vi "PictureControlGUIForMissingClasses.vi"() -> ()   [LabVIEW 2016]
uses:
  <vilib>/picture/picture.llb/imagedata.ctl
  <vilib>/Utility/miscctls.llb/LVFontTypeDef.ctl
  <vilib>/Utility/miscctls.llb/LVBoundsTypeDef.ctl
panel:
  in  "Items":T1(array[cluster])=[{"Item"="IDisposne", "Options"=["Select action to handle missing type", "Create stub code as class", "Create stub code as interface by aggregation", "Create stub code as interface by VI Serevr", "Remove dependency to this type"], "Icons"=[enum."?", enum."Add", enum."Add", enum."Add", enum."Delete"], "InitialIndex"=0}, {"Item"="IInterafceXXX", "Options"=["Select action to handle missing type", "Create stub code as class", "Create stub code as interface by VI Serevr", "Remove dependency to this type"], "Icons"=[enum."?", enum."Add", enum."Add", enum."Delete"], "InitialIndex"=1}, {"Item"="Something Something", "Options"=["Select action to handle missing type", "Create stub code as class", "Remove dependency to this type"], "Icons"=[enum."?", enum."Add", enum."Delete"], "InitialIndex"=2}, {"Item"="Something Something", "Options"=["Select action to handle missing type", "Create stub code as class", "Remove dependency to this type"], "Icons"=[enum."?", enum."Add", enum."Delete"], "InitialIndex"=2}, {"Item"="Something Something", "Options"=["Select action to handle missing type", "Create stub code as class", "Remove dependency to this type"], "Icons"=[enum."?", enum."Add", enum."Delete"], "InitialIndex"=2}, {"Item"="Something Something", "Options"=["Select action to handle missing type", "Create stub code as class", "Remove dependency to this type"], "Icons"=[enum."?", enum."Add", enum."Delete"], "InitialIndex"=2}, {"Item"="Something Something", "Options"=["Select action to handle missing type", "Create stub code as class", "Remove dependency to this type"], "Icons"=[enum."?", enum."Add", enum."Delete"], "InitialIndex"=2}, {"Item"="Something Something", "Options"=["Select action to handle missing type", "Create stub code as class", "Remove dependency to this type"], "Icons"=[enum."?", enum."Add", enum."Delete"], "InitialIndex"=2}]
  out "Mouse Position":cluster{"X":i32, "Y":i32}={"X"=267, "Y"=20}
  in  "Ring":u16(ring)=2 items=["Select action to handle missing type", "Create stub code as class", "Remove dependency to this type"]
  out "Picture":picture caption="Missing Classes and types"
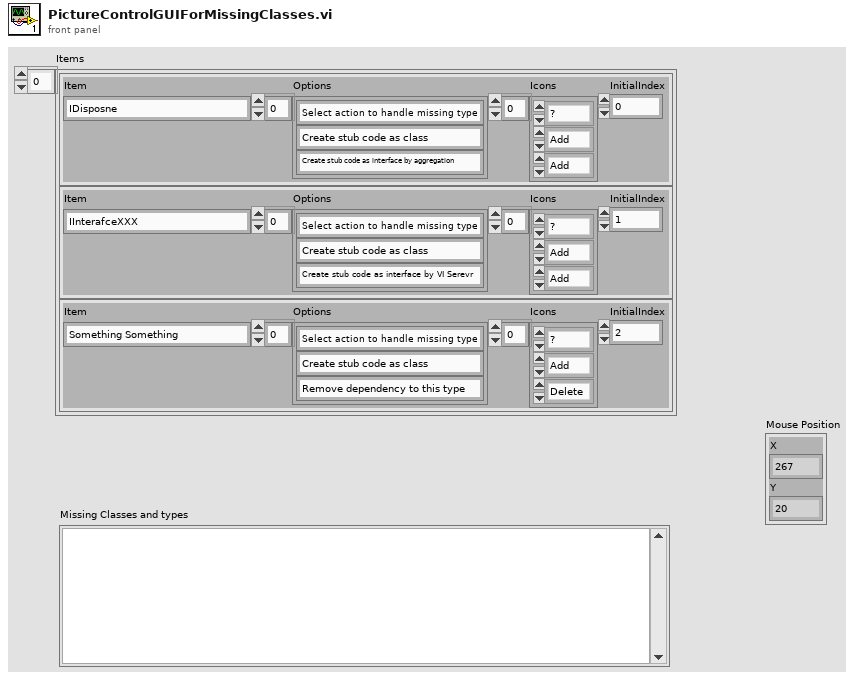
[diagram p1: front panel]
types:
  T1 = cluster{"Item":string, "Options":string[], "Icons":enum16{"?", "Add", "Delete"}[], "InitialIndex":i32}[]
  T2 = typedef "imagedata.ctl" = cluster{"image type":i32, "image depth":i32, "image":u8[], "mask":u8[], "colors":u32[], "Rectangle":cluster{"left":i16, "top":i16, "right":i16, "bottom":i16}}
  T3 = cluster{"ShowRing":bool, "Rectangle":cluster{"left":i16, "top":i16, "right":i16, "bottom":i16}, "IndexOffset":i32, "Row":i32, "Y-Distance":i32, "Selected":i32[], "Font":enum16{"User-specified Font", "Application Font", "System Font", "Dialog Font"}, "UserFont":cluster{"Font Name:":string, "Size":i16, "Strikeout?":bool, "Italic?":bool, "Underline?":bool, "Outline?":bool, "Shadow?":bool, "Bold?":bool}, "VerGap":i32, "HorGap":i32, "XStart2":i32, "XStart1":i32, "Rectangles":cluster{"left":i16, "top":i16, "right":i16, "bottom":i16}[], "VerticalRows":i32, "YStart":i32}
  T4 = typedef "LVFontTypeDef.ctl" = cluster{"Font Name":string, "Size":u16, "Bold":bool, "Italic":bool, "Underline":bool, "Strikeout":bool, "Color":u32}
  T5 = cluster{"left":i16, "top":i16, "right":i16, "bottom":i16}
  T6 = typedef "LVBoundsTypeDef.ctl" = cluster{"Width":u32, "Height":u32}
  T7 = cluster{"Font Name:":string, "Size":i16, "Strikeout?":bool, "Italic?":bool, "Underline?":bool, "Outline?":bool, "Shadow?":bool, "Bold?":bool}
  T8 = enum16{"User-specified Font", "Application Font", "System Font", "Dialog Font"}
  T9 = typedef "LVMouseTypeDef.ctl" = cluster{"Mouse Position":cluster{"X":i32, "Y":i32}, "Mouse Modifiers":cluster{"Button Down":bool, "Shift Mod":bool, "Menu Mod":bool, "Option Mod":bool}}
  T10 = cluster{"left":i16, "top":i16, "right":i16, "bottom":i16}[]
  T11 = cluster{"Item":string, "Options":string[], "Icons":enum16{"?", "Add", "Delete"}[], "InitialIndex":i32}
  T12 = typedef "LVRectTypeDef.ctl" = cluster{"Left":i16, "Top":i16, "Right":i16, "Bottom":i16}
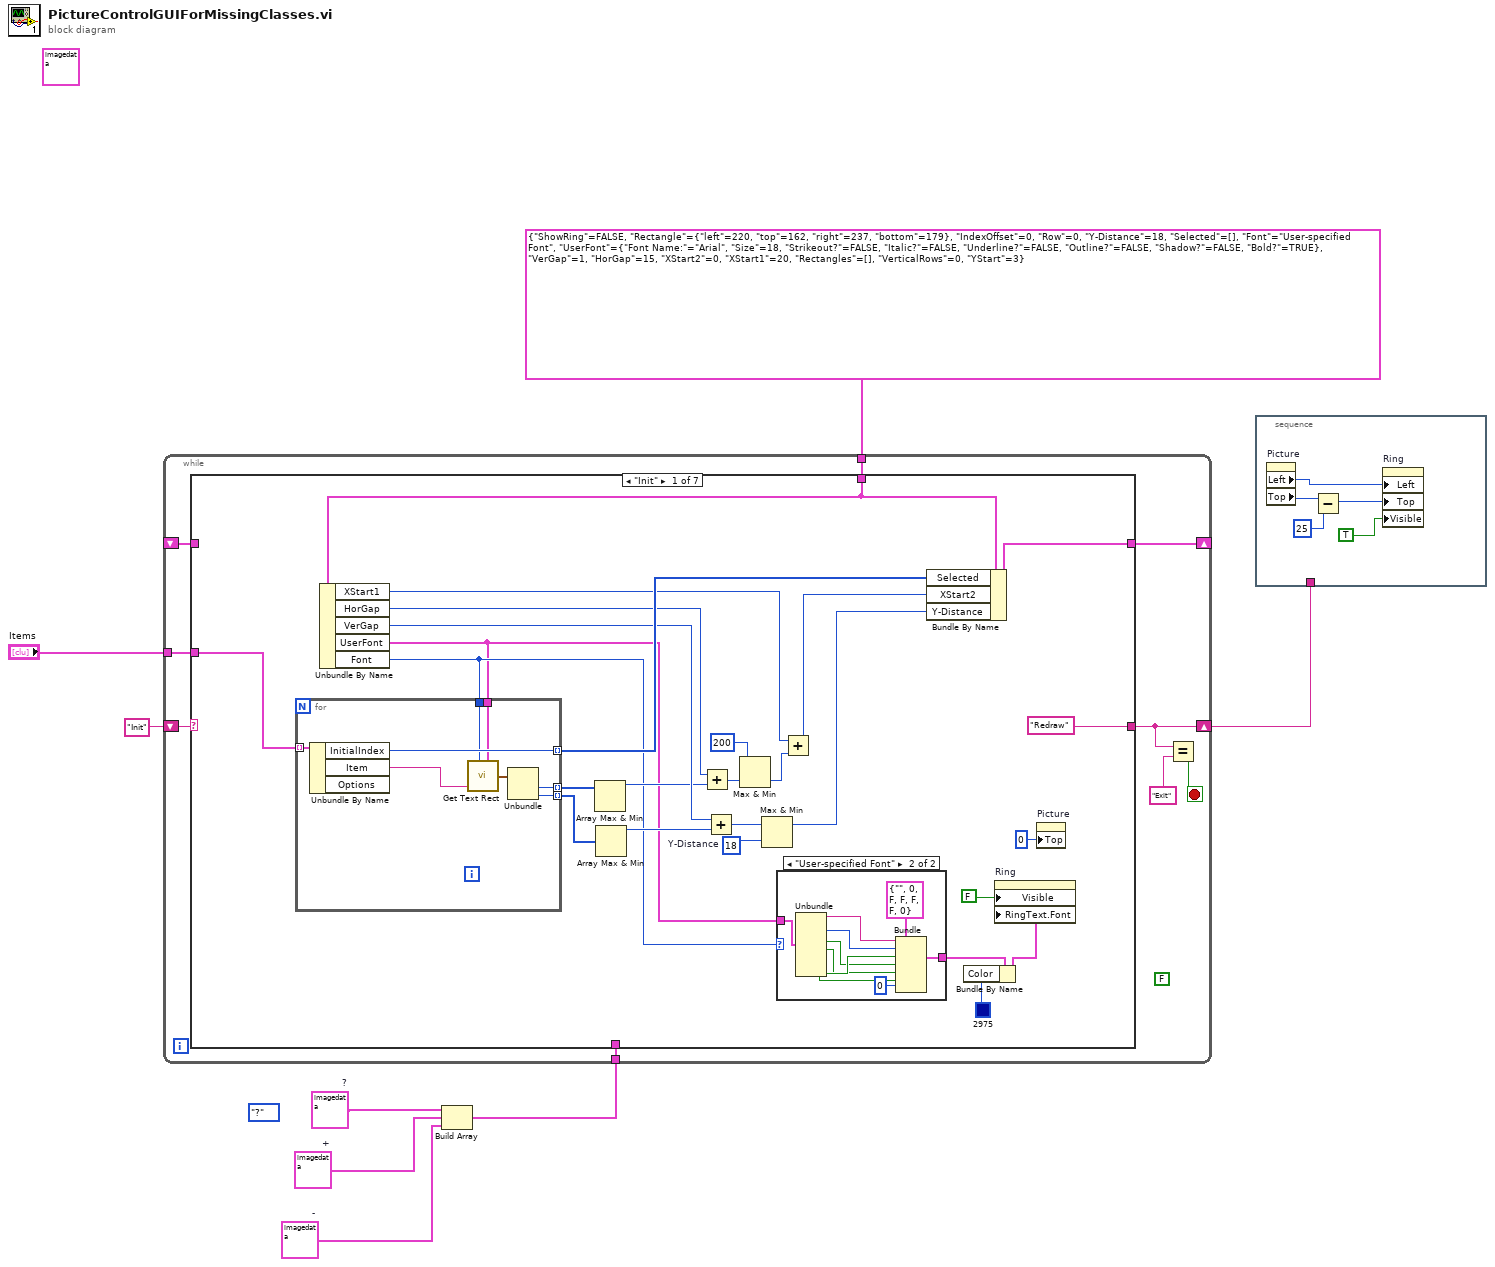
[diagram p0: block diagram]
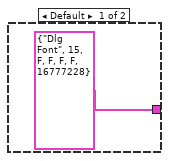
[diagram p2: hidden frame]
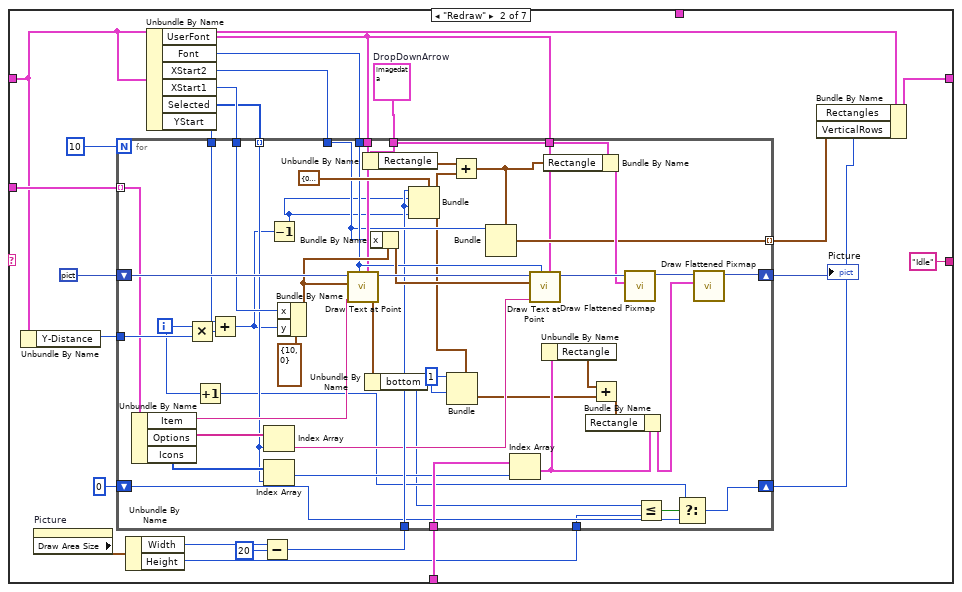
[diagram p3: hidden frame]
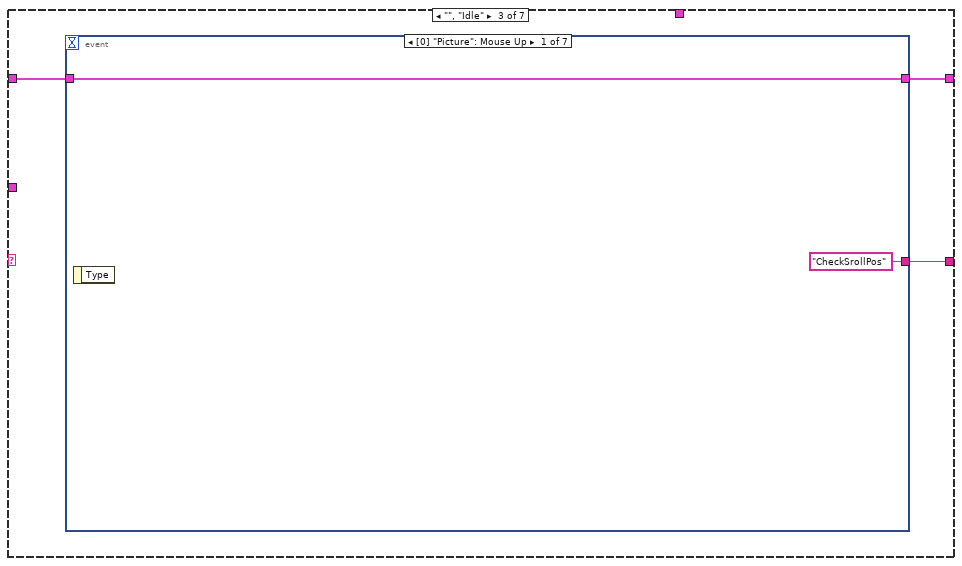
[diagram p4: hidden frame]
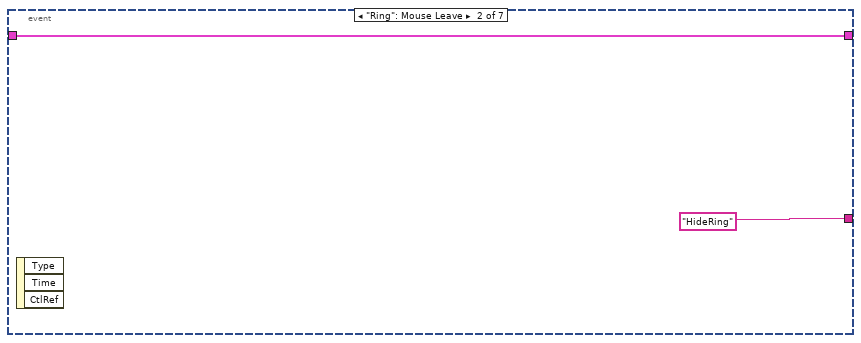
[diagram p5: hidden frame]
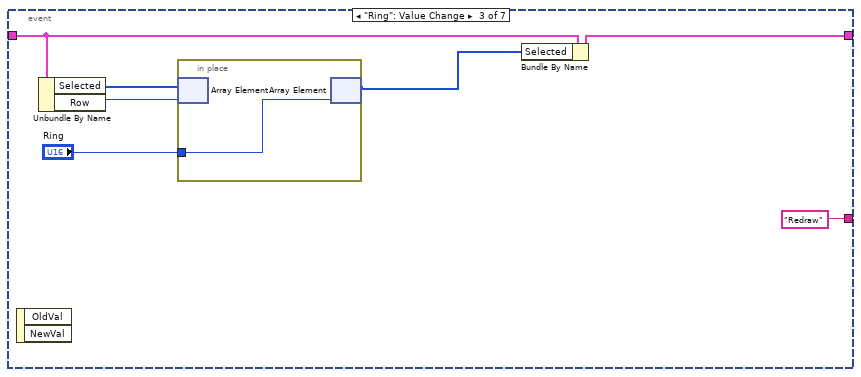
[diagram p6: hidden frame]
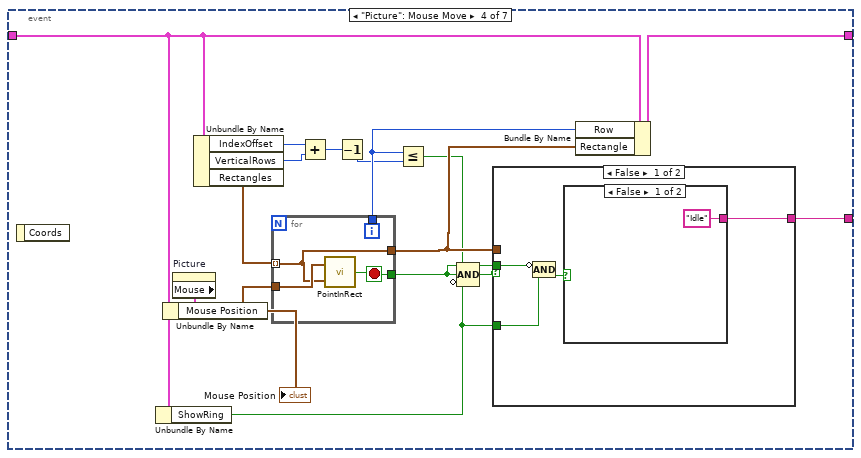
[diagram p7: hidden frame]
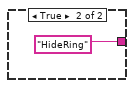
[diagram p8: hidden frame]
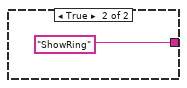
[diagram p9: hidden frame]
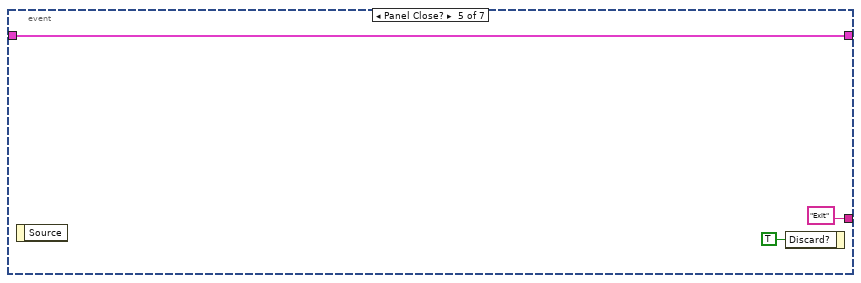
[diagram p10: hidden frame]
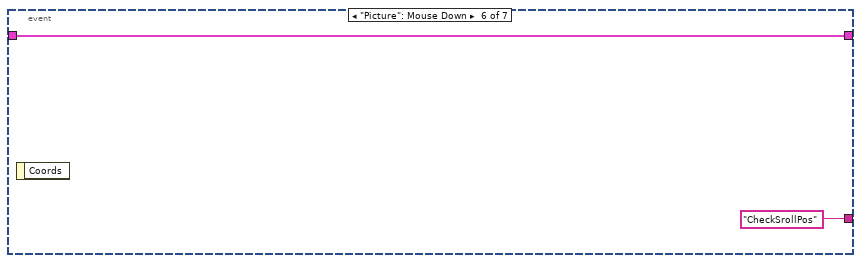
[diagram p11: hidden frame]
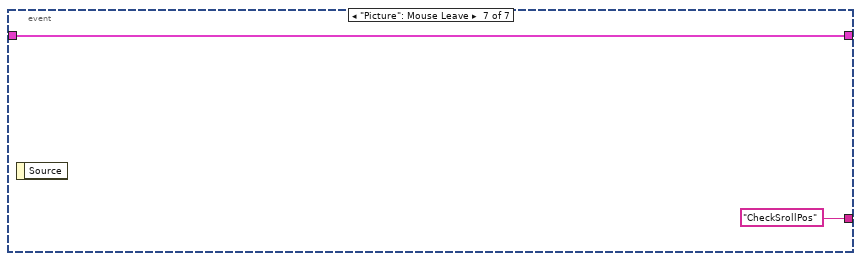
[diagram p12: hidden frame]
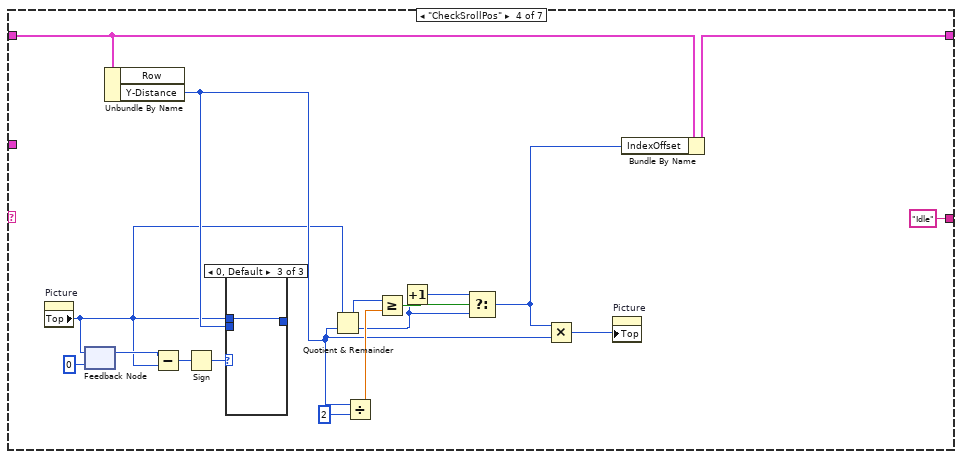
[diagram p13: hidden frame]
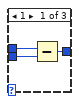
[diagram p14: hidden frame]
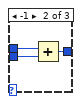
[diagram p15: hidden frame]
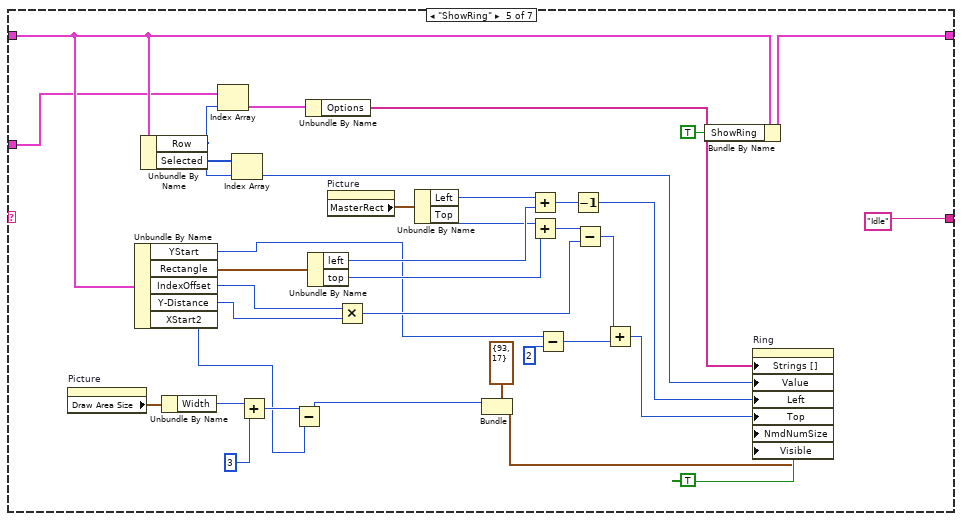
[diagram p16: hidden frame]
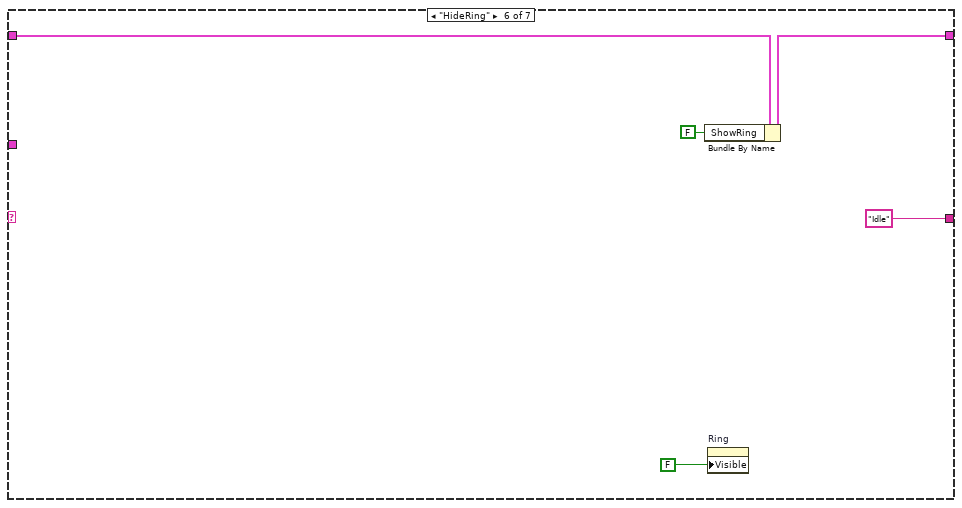
[diagram p17: hidden frame]
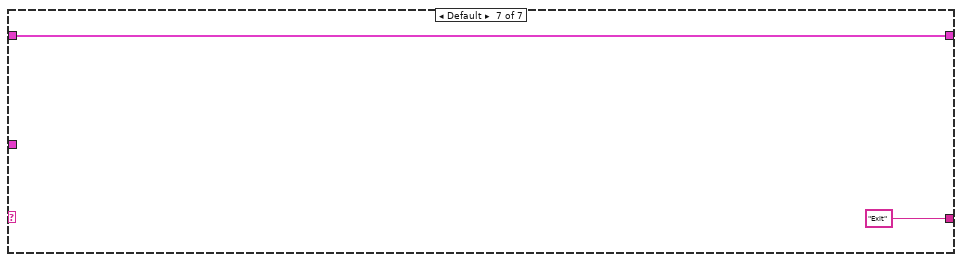
[diagram p18: hidden frame]
diagram:
  (unwired) enum16{"?", "Add", "Delete"}."?" ("element")
  w3 = T2 {"image type"=0, "image depth"=32, "image"=array[1024 elements], "mask"=[0, 0, 15, 224, 63, 248, 127, 252, 127, 252, 255, 254, 255, 254, 255, 254, 255, 254, 255, 254, 255, 254, 255, 254, 127, 252, 127, 252, 63, 248, 15, 224], "colors"=[], "Rectangle"={"left"=0, "top"=0, "right"=16, "bottom"=16}}  # ?
  w1 = T2 {"image type"=0, "image depth"=32, "image"=[0, 0, 0, 0, 0, 0, 0, 0, 78, 142, 77, 90, 2, 148, 148, 147, 0, 0, 0, 0, 0, 0, 0, 0, 0, 0, 0, 0, 0, 0, 0, 0, 0, 0, 0, 0, 0, 0, 0, 0, 0, 0, 0, 0, 48, 145, 103, 111, 3, 148, 145, 146, 0, 0, 0, 0, 0, 0, 0, 0, 0, 0, 0, 0, 0, 0, 0, 0, 113, 246, 155, 172, 255, 238, 54, 90, 164, 243, 121, 144, 0, 0, 0, 0, 0, 0, 0, 0, 0, 0, 0, 0, 0, 0, 0, 0, 0, 0, 0, 0, 0, 0, 0, 0, 114, 247, 158, 175, 255, 238, 55, 91, 247, 238, 61, 95, 190, 242, 101, 128, 55, 251, 205, 215, 0, 0, 0, 0, 37, 251, 214, 220, 252, 236, 52, 88, 255, 237, 57, 92, 255, 235, 54, 90, 150, 242, 130, 151, 0, 0, 0, 0, 0, 0, 0, 0, 0, 0, 0, 0, 0, 0, 0, 0, 64, 249, 199, 209, 253, 236, 55, 90, 254, 235, 56, 91, 255, 236, 54, 90, 127, 244, 146, 165, 0, 0, 0, 0, 0, 0, 0, 0, 0, 0, 0, 0, 64, 249, 193, 203, 240, 236, 60, 95, 255, 237, 57, 92, 255, 236, 55, 90, 136, 243, 141, 161, 0, 0, 0, 0, 0, 0, 0, 0, 25, 252, 231, 235, 235, 237, 66, 99, 255, 236, 57, 92, 255, 236, 54, 90, 118, 244, 150, 168, 0, 0, 0, 0, 0, 0, 0, 0, 0, 0, 0, 0, 0, 0, 0, 0, 0, 0, 0, 0, 39, 251, 215, 222, 224, 237, 70, 103, 255, 236, 57, 92, 255, 235, 53, 89, 121, 244, 152, 170, 1, 254, 253, 254, 201, 239, 91, 120, 254, 235, 56, 91, 255, 236, 55, 90, 121, 244, 150, 168, 0, 0, 0, 0, 0, 0, 0, 0, 0, 0, 0, 0, 0, 0, 0, 0, 0, 0, 0, 0, 0, 0, 0, 0, 0, 0, 0, 0, 20, 252, 233, 236, 204, 238, 86, 115, 255, 236, 57, 92, 255, 236, 55, 91, 194, 239, 93, 122, 255, 236, 56, 92, 255, 236, 55, 90, 133, 243, 143, 163, 0, 0, 0, 0, 0, 0, 0, 0, 0, 0, 0, 0, 0, 0, 0, 0, 0, 0, 0, 0, 0, 0, 0, 0, 0, 0, 0, 0, 0, 0, 0, 0, 0, 0, 0, 0, 12, 253, 243, 245, 210, 238, 83, 114, 255, 236, 57, 92, 254, 235, 56, 91, 255, 236, 56, 92, 149, 242, 132, 153, 0, 0, 0, 0, 0, 0, 0, 0, 0, 0, 0, 0, 0, 0, 0, 0, 0, 0, 0, 0, 0, 0, 0, 0, 0, 0, 0, 0, 0, 0, 0, 0, 0, 0, 0, 0, 0, 0, 0, 0, 0, 0, 0, 0, 78, 248, 186, 198, 255, 236, 55, 91, 255, 237, 58, 93, 253, 236, 55, 90, 39, 251, 220, 226, 0, 0, 0, 0, 0, 0, 0, 0, 0, 0, 0, 0, 0, 0, 0, 0, 0, 0, 0, 0, 0, 0, 0, 0, 0, 0, 0, 0, 0, 0, 0, 0, 0, 0, 0, 0, 0, 0, 0, 0, 11, 253, 244, 245, 222, 237, 74, 105, 254, 236, 56, 92, 253, 236, 56, 91, 255, 236, 57, 92, 210, 238, 85, 116, 5, 254, 250, 250, 0, 0, 0, 0, 0, 0, 0, 0, 0, 0, 0, 0, 0, 0, 0, 0, 0, 0, 0, 0, 0, 0, 0, 0, 0, 0, 0, 0, 0, 0, 0, 0, 0, 0, 0, 0, 167, 241, 117, 142, 255, 236, 55, 91, 179, 240, 108, 134, 139, 244, 138, 159, 255, 236, 56, 91, 255, 236, 56, 91, 147, 243, 132, 153, 0, 0, 0, 0, 0, 0, 0, 0, 0, 0, 0, 0, 0, 0, 0, 0, 0, 0, 0, 0, 0, 0, 0, 0, 0, 0, 0, 0, 0, 0, 0, 0, 100, 247, 169, 184, 255, 236, 55, 90, 255, 235, 54, 90, 54, 250, 206, 215, 6, 253, 248, 249, 227, 237, 71, 103, 254, 235, 56, 91, 255, 236, 54, 90, 77, 248, 188, 200, 0, 0, 0, 0, 0, 0, 0, 0, 0, 0, 0, 0, 0, 0, 0, 0, 0, 0, 0, 0, 0, 0, 0, 0, 40, 251, 219, 224, 247, 236, 57, 92, 255, 236, 57, 92, 185, 240, 103, 129, 0, 0, 0, 0, 0, 0, 0, 0, 100, 246, 164, 180, 255, 236, 56, 91, 255, 236, 57, 92, 238, 237, 64, 98, 25, 252, 232, 236, 0, 0, 0, 0, 0, 0, 0, 0, 0, 0, 0, 0, 0, 0, 0, 0, 4, 254, 250, 251, 211, 238, 83, 113, 254, 235, 56, 91, 255, 236, 54, 90, 56, 250, 206, 214, 0, 0, 0, 0, 0, 0, 0, 0, 4, 254, 247, 249, 228, 237, 68, 100, 255, 237, 57, 92, 254, 235, 56, 91, 193, 239, 96, 125, 0, 0, 0, 0, 0, 0, 0, 0, 0, 0, 0, 0, 0, 0, 0, 0, 139, 244, 137, 157, 255, 237, 55, 91, 255, 237, 56, 92, 188, 229, 93, 119, 0, 0, 0, 0, 0, 0, 0, 0, 0, 0, 0, 0, 0, 0, 0, 0, 105, 246, 160, 177, 255, 236, 55, 90, 255, 236, 56, 92, 255, 236, 54, 90, 127, 244, 148, 166, 0, 0, 0, 0, 0, 0, 0, 0, 26, 246, 224, 228, 199, 228, 84, 112, 200, 227, 87, 114, 201, 227, 85, 113, 57, 237, 196, 204, 0, 0, 0, 0, 0, 0, 0, 0, 0, 0, 0, 0, 0, 0, 0, 0, 7, 254, 247, 249, 171, 231, 108, 133, 170, 241, 120, 144, 167, 239, 120, 143, 162, 235, 117, 140, 17, 241, 227, 230, 0, 0, 0, 0, 0, 0, 0, 0, 0, 0, 0, 0, 0, 0, 0, 0, 0, 0, 0, 0, 0, 0, 0, 0, 0, 0, 0, 0, 0, 0, 0, 0, 0, 0, 0, 0, 0, 0, 0, 0, 0, 0, 0, 0, 0, 0, 0, 0, 0, 0, 0, 0, 0, 0, 0, 0, 0, 0, 0, 0, 0, 0, 0, 0, 0, 0, 0, 0], "mask"=[0, 0, 48, 28, 120, 60, 60, 112, 28, 224, 15, 224, 7, 192, 3, 128, 7, 192, 15, 224, 12, 224, 28, 112, 56, 120, 120, 60, 112, 60, 0, 0], "colors"=[], "Rectangle"={"left"=0, "top"=0, "right"=16, "bottom"=16}}  # -
  w2 = T2 {"image type"=0, "image depth"=32, "image"=[0, 0, 0, 0, 0, 0, 0, 0, 0, 0, 0, 0, 0, 0, 0, 0, 0, 0, 0, 0, 255, 0, 173, 0, 255, 0, 173, 0, 255, 0, 173, 0, 255, 0, 173, 0, 255, 0, 173, 0, 0, 0, 0, 0, 0, 0, 0, 0, 0, 0, 0, 0, 0, 0, 0, 0, 0, 0, 0, 0, 0, 0, 0, 0, 0, 0, 0, 0, 0, 0, 0, 0, 0, 0, 0, 0, 0, 0, 0, 0, 0, 0, 0, 0, 255, 0, 173, 0, 255, 0, 173, 0, 255, 0, 173, 0, 255, 0, 173, 0, 255, 0, 173, 0, 255, 106, 100, 106, 0, 0, 0, 0, 0, 0, 0, 0, 0, 0, 0, 0, 0, 0, 0, 0, 0, 0, 0, 0, 0, 0, 0, 0, 0, 0, 0, 0, 0, 0, 0, 0, 0, 0, 0, 0, 0, 0, 0, 0, 255, 0, 173, 0, 255, 0, 173, 0, 255, 0, 173, 0, 255, 0, 173, 0, 255, 0, 173, 0, 255, 106, 100, 106, 0, 0, 0, 0, 0, 0, 0, 0, 0, 0, 0, 0, 0, 0, 0, 0, 0, 0, 0, 0, 0, 0, 0, 0, 0, 0, 0, 0, 0, 0, 0, 0, 0, 0, 0, 0, 0, 0, 0, 0, 255, 0, 173, 0, 255, 0, 173, 0, 255, 0, 173, 0, 255, 0, 173, 0, 255, 0, 173, 0, 255, 106, 100, 106, 0, 0, 0, 0, 0, 0, 0, 0, 0, 0, 0, 0, 0, 0, 0, 0, 0, 0, 0, 0, 0, 0, 0, 0, 0, 0, 0, 0, 0, 0, 0, 0, 0, 0, 0, 0, 0, 0, 0, 0, 255, 0, 173, 0, 255, 0, 173, 0, 255, 0, 173, 0, 255, 0, 173, 0, 255, 0, 173, 0, 255, 106, 100, 106, 0, 0, 0, 0, 0, 0, 0, 0, 0, 0, 0, 0, 0, 0, 0, 0, 0, 0, 0, 0, 255, 0, 173, 0, 255, 0, 173, 0, 255, 0, 173, 0, 255, 0, 173, 0, 255, 0, 173, 0, 255, 0, 173, 0, 255, 0, 173, 0, 255, 0, 173, 0, 255, 0, 173, 0, 255, 0, 173, 0, 255, 0, 173, 0, 255, 0, 173, 0, 255, 0, 173, 0, 255, 0, 173, 0, 255, 0, 173, 0, 0, 0, 0, 0, 255, 0, 173, 0, 255, 0, 173, 0, 255, 0, 173, 0, 255, 0, 173, 0, 255, 0, 173, 0, 255, 0, 173, 0, 255, 0, 173, 0, 255, 0, 173, 0, 255, 0, 173, 0, 255, 0, 173, 0, 255, 0, 173, 0, 255, 0, 173, 0, 255, 0, 173, 0, 255, 0, 173, 0, 255, 0, 173, 0, 255, 106, 100, 106, 255, 0, 173, 0, 255, 0, 173, 0, 255, 0, 173, 0, 255, 0, 173, 0, 255, 0, 173, 0, 255, 0, 173, 0, 255, 0, 173, 0, 255, 0, 173, 0, 255, 0, 173, 0, 255, 0, 173, 0, 255, 0, 173, 0, 255, 0, 173, 0, 255, 0, 173, 0, 255, 0, 173, 0, 255, 0, 173, 0, 255, 106, 100, 106, 255, 0, 173, 0, 255, 0, 173, 0, 255, 0, 173, 0, 255, 0, 173, 0, 255, 0, 173, 0, 255, 0, 173, 0, 255, 0, 173, 0, 255, 0, 173, 0, 255, 0, 173, 0, 255, 0, 173, 0, 255, 0, 173, 0, 255, 0, 173, 0, 255, 0, 173, 0, 255, 0, 173, 0, 255, 0, 173, 0, 255, 106, 100, 106, 255, 0, 173, 0, 255, 0, 173, 0, 255, 0, 173, 0, 255, 0, 173, 0, 255, 0, 173, 0, 255, 0, 173, 0, 255, 0, 173, 0, 255, 0, 173, 0, 255, 0, 173, 0, 255, 0, 173, 0, 255, 0, 173, 0, 255, 0, 173, 0, 255, 0, 173, 0, 255, 0, 173, 0, 255, 0, 173, 0, 255, 106, 100, 106, 0, 0, 0, 0, 255, 106, 100, 106, 255, 106, 100, 106, 255, 106, 100, 106, 255, 106, 100, 106, 255, 0, 173, 0, 255, 0, 173, 0, 255, 0, 173, 0, 255, 0, 173, 0, 255, 0, 173, 0, 255, 106, 100, 106, 255, 106, 100, 106, 255, 106, 100, 106, 255, 106, 100, 106, 255, 106, 100, 106, 255, 106, 100, 106, 0, 0, 0, 0, 0, 0, 0, 0, 0, 0, 0, 0, 0, 0, 0, 0, 0, 0, 0, 0, 255, 0, 173, 0, 255, 0, 173, 0, 255, 0, 173, 0, 255, 0, 173, 0, 255, 0, 173, 0, 255, 106, 100, 106, 0, 0, 0, 0, 0, 0, 0, 0, 0, 0, 0, 0, 0, 0, 0, 0, 0, 0, 0, 0, 0, 0, 0, 0, 0, 0, 0, 0, 0, 0, 0, 0, 0, 0, 0, 0, 0, 0, 0, 0, 255, 0, 173, 0, 255, 0, 173, 0, 255, 0, 173, 0, 255, 0, 173, 0, 255, 0, 173, 0, 255, 106, 100, 106, 0, 0, 0, 0, 0, 0, 0, 0, 0, 0, 0, 0, 0, 0, 0, 0, 0, 0, 0, 0, 0, 0, 0, 0, 0, 0, 0, 0, 0, 0, 0, 0, 0, 0, 0, 0, 0, 0, 0, 0, 255, 0, 173, 0, 255, 0, 173, 0, 255, 0, 173, 0, 255, 0, 173, 0, 255, 0, 173, 0, 255, 106, 100, 106, 0, 0, 0, 0, 0, 0, 0, 0, 0, 0, 0, 0, 0, 0, 0, 0, 0, 0, 0, 0, 0, 0, 0, 0, 0, 0, 0, 0, 0, 0, 0, 0, 0, 0, 0, 0, 0, 0, 0, 0, 255, 0, 173, 0, 255, 0, 173, 0, 255, 0, 173, 0, 255, 0, 173, 0, 255, 0, 173, 0, 255, 106, 100, 106, 0, 0, 0, 0, 0, 0, 0, 0, 0, 0, 0, 0, 0, 0, 0, 0, 0, 0, 0, 0, 0, 0, 0, 0, 0, 0, 0, 0, 0, 0, 0, 0, 0, 0, 0, 0, 0, 0, 0, 0, 0, 0, 0, 0, 255, 106, 100, 106, 255, 106, 100, 106, 255, 106, 100, 106, 255, 106, 100, 106, 255, 106, 100, 106, 0, 0, 0, 0, 0, 0, 0, 0, 0, 0, 0, 0, 0, 0, 0, 0, 0, 0, 0, 0], "mask"=[7, 192, 7, 224, 7, 224, 7, 224, 7, 224, 255, 254, 255, 255, 255, 255, 255, 255, 255, 255, 127, 255, 7, 224, 7, 224, 7, 224, 7, 224, 3, 224], "colors"=[], "Rectangle"={"left"=0, "top"=0, "right"=16, "bottom"=16}}  # +
  (unwired) T2 {"image type"=0, "image depth"=32, "image"=array[1156 elements], "mask"=[255, 255, 128, 0, 255, 255, 128, 0, 255, 255, 128, 0, 255, 255, 128, 0, 255, 255, 128, 0, 255, 255, 128, 0, 255, 255, 128, 0, 255, 255, 128, 0, 255, 255, 128, 0, 255, 255, 128, 0, 255, 255, 128, 0, 255, 255, 128, 0, 255, 255, 128, 0, 255, 255, 128, 0, 255, 255, 128, 0, 255, 255, 128, 0, 255, 255, 128, 0], "colors"=[], "Rectangle"={"left"=0, "top"=0, "right"=17, "bottom"=17}} ("image data")
  n1 = Build Array(w3, w2, w1) -> (w4:T2[])
  n2 = while {
    shift-right: [w14] -> w5
    shift-left: "Init" ("format string") -> [w17]
    shift-right: [w16] -> _
    shift-left: _ -> [w15]
    tunnel: "Items" -> [w11]
    tunnel: T3 {"ShowRing"=FALSE, "Rectangle"={"left"=220, "top"=162, "right"=237, "bottom"=179}, "IndexOffset"=0, "Row"=0, "Y-Distance"=18, "Selected"=[], "Font"=enum."User-specified Font", "UserFont"={"Font Name:"="Arial", "Size"=18, "Strikeout?"=FALSE, "Italic?"=FALSE, "Underline?"=FALSE, "Outline?"=FALSE, "Shadow?"=FALSE, "Bold?"=TRUE}, "VerGap"=1, "HorGap"=15, "XStart2"=0, "XStart1"=20, "Rectangles"=[], "VerticalRows"=0, "YStart"=3} -> [w10]
    tunnel: w4 -> [w9]
    stop <- w12 stop-if-true
    (unwired) FALSE
    n3 = case shown="\"Init\"" w17 {
      tunnel: ["Redraw" ("format string") "Idle" ("format string") w137 "Idle" ("format string") "Idle" ("format string") "Idle" ("format string") "Exit" ("format string")] -> w14
      tunnel: [w39 w79 w135 w191 w238 w247 w250] -> w16
      tunnel: w15 -> [_ w77 w136 w192 w229 w248 w250]
      tunnel: w11 -> [w40 w82 _ _ w227 _ _]
      tunnel: w10 -> [w37 _ _ _ _ _ _]
      tunnel: w9 -> [_ w67 _ _ _ _ _]
      frame "Init" {
        w34 = 18  # Y-Distance
        n4 = Unbundle By Name(w37) -> ("XStart1"=w24:i32, "HorGap"=w28:i32, "VerGap"=w30:i32, "UserFont"=w20:T7, "Font"=w21:T8)
        n5 = for {
          tunnel: w40 -> [w62] mode=indexing
          tunnel: [w61] -> w38 mode=indexing
          tunnel: w21 -> [w60]
          tunnel: w20 -> [w59]
          tunnel: [w57] -> w36 mode=indexing
          tunnel: [w56] -> w35 mode=indexing
          n6 = Unbundle By Name(w62) -> ("InitialIndex"=w61:i32, "Item"=w55:string)  [unwired: 1 out]
          n7 = call <vilib>:"Get Text Rect.vi"("desired font(Application)"=w60, "text"=w55, "[user-specified font]"=w59) -> ("rect"=w58:T5)  [unwired: 6 in]
          n8 = Unbundle(w58) -> ("right"=w57:i16, "bottom"=w56:i16)  [unwired: 2 out]
        }
        n9 = Array Max & Min(array=w36) -> (max value=w29:i16)  [unwired: 3 out]
        n10 = Array Max & Min(array=w35) -> (max value=w33:i16)  [unwired: 3 out]
        n11 = Add(x=w28, y=w29) -> (x+y=w27:i32)
        n12 = Add(x=w30, y=w33) -> (x+y=w32:i32)
        n13 = Max & Min(x=200, y=w27) -> (min(x,y)=w25:i32)  [unwired: 1 out]
        n14 = Max & Min(x=w32, y=w34) -> (max(x,y)=w31:i32)  [unwired: 1 out]
        n15 = case shown="\"User-specified Font\"" w21 {
          tunnel: [T4 {"Font Name"="Dlg Font", "Size"=15, "Bold"=FALSE, "Italic"=FALSE, "Underline"=FALSE, "Strikeout"=FALSE, "Color"=16777228} ("Ring Text.Font") w53] -> w22
          tunnel: w20 -> [_ w52]
          frame Default {
          }
          frame "User-specified Font" {
            n16 = Unbundle(w52) -> ("Font Name:"=w51:string, "Size"=w50:i16, "Strikeout?"=w46:bool, "Italic?"=w48:bool, "Underline?"=w47:bool, "Bold?"=w49:bool)  [unwired: 2 out]
            n17 = Bundle(cluster=T4 {"Font Name"="", "Size"=0, "Bold"=FALSE, "Italic"=FALSE, "Underline"=FALSE, "Strikeout"=FALSE, "Color"=0} ("Ring Text.Font"), "Font Name"=w51, "Size"=w50, "Bold"=w49, "Italic"=w48, "Underline"=w47, "Strikeout"=w46, "Color"=u32 0) -> (w53:T4)
          }
        }
        n18 = Add(x=w24, y=w25) -> (x+y=w23:i32)
        n19 = Bundle By Name(cluster=w37, "Selected"=w38, "XStart2"=w23, "Y-Distance"=w31) -> (w39:T3)
        n20 = Bundle By Name(cluster=w22, "Color"=u32 2975) -> (w19:T4)
        n21 = property on="Ring" class="Ring (strict)"("Visible"=FALSE, "RingText.Font"=w19) -> ()  [unwired: 2 in, 2 out]
        n22 = property on="Picture" class="Pict"("Top"=i16 0 ("Origin:Top")) -> ()  [unwired: 2 in, 2 out]
      }
      frame "Redraw" {
        w86 = T2 {"image type"=0, "image depth"=24, "image"=array[867 elements], "mask"=[], "colors"=[], "Rectangle"={"left"=0, "top"=0, "right"=17, "bottom"=17}}  # DropDownArrow
        n23 = Unbundle By Name(w77) -> ("Y-Distance"=w81:i32)
        n24 = property on="Picture" class="Pict"() -> ("Draw Area Size"=w72:T6)  [unwired: 2 in, 2 out]
        n25 = Unbundle By Name(w72) -> ("Width"=w71:u32, "Height"=w63:u32)
        n26 = Unbundle By Name(w77) -> ("UserFont"=w75:T7, "Font"=w76:T8, "XStart2"=w73:i32, "XStart1"=w74:i32, "Selected"=w69:i32[], "YStart"=w68:i32)
        n27 = Subtract(x=w71, y=u32 20) -> (x-y=w65:u32)
        n28 = for {
          N: 10 -> [_]
          shift-right: [w106] -> w85
          shift-left: picture data[5B] ("new picture") -> [w134]
          tunnel: w86 -> [w127]
          tunnel: w81 -> [w122]
          tunnel: w82 -> [w120] mode=indexing
          tunnel: [w119] -> w78 mode=indexing
          tunnel: w76 -> [w118]
          tunnel: w75 -> [w117]
          tunnel: w75 -> [w116]
          tunnel: w74 -> [w115]
          tunnel: w73 -> [w114]
          tunnel: w65 -> [w113]
          tunnel: w69 -> [w104] mode=indexing
          tunnel: w68 -> [w109]
          tunnel: w67 -> [w103]
          shift-right: [w91] -> w64
          shift-left: 0 -> [w90]
          tunnel: w63 -> [w87]
          i -> [w121]
          w95 = i16 1 ("left")
          n29 = Unbundle By Name(w120) -> ("Item"=w110:string, "Options"=w112:string[], "Icons"=w105:enum16{"?", "Add", "Delete"}[])
          n30 = Multiply(x=w121, y=w122) -> (x*y=w124:i32)
          n31 = Increment(x=w121) -> (x+1=w93:i32)
          n32 = Add(x=w109, y=w124) -> (x+y=w92:i32)
          n33 = Index Array(array=w112, index=w104) -> (element=w111:string)
          n34 = Index Array(array=w105, index=w104) -> (element=w102:enum16{"?", "Add", "Delete"})
          n35 = Decrement(x=w92) -> (x-1=w108:i32)
          n36 = Bundle By Name(cluster=cluster{"x":i16, "y":i16} {"x"=10, "y"=0} ("origin"), "x"=w115, "y"=w92) -> (w131:cluster{"x":i16, "y":i16})
          n37 = call <vilib>:"Draw Text at Point.vi"("[user-specified font]"=w117, "desired font(Application)"=w118, "text"=w110, "origin"=w131, "picture"=w134) -> ("text rect"=w89:T5, "new picture"=w132:picture)  [unwired: 5 in]
          n38 = Unbundle By Name(w127) -> ("Rectangle"=w128:T5)
          n39 = Unbundle By Name(w89) -> ("bottom"=w88:i16)
          n40 = Bundle By Name(cluster=w131, "x"=w114) -> (w130:cluster{"x":i16, "y":i16})
          n41 = Bundle(cluster=T5 {"left"=0, "top"=0, "right"=0, "bottom"=0} ("y"), "left"=w113, "top"=w108, "right"=w113, "bottom"=w108) -> (w97:T5)
          n42 = Bundle(cluster=w97, "left"=w95, "right"=w95) -> (w96:T5)  [unwired: 2 in]
          n43 = Add(x=w128, y=w97) -> (x+y=w123:T5)
          n44 = Bundle(cluster=w123, "left"=w114) -> (w119:T5)  [unwired: 3 in]
          n45 = Index Array(array=w103, index=w102) -> (element=w100:T2)
          n46 = call <vilib>:"Draw Text at Point.vi"("[user-specified font]"=w116, "desired font(Application)"=w118, "text"=w111, "origin"=w130, "picture"=w132) -> ("new picture"=w129:picture)  [unwired: 5 in, 1 out]
          n47 = Unbundle By Name(w100) -> ("Rectangle"=w99:T5)
          n48 = Bundle By Name(cluster=w127, "Rectangle"=w123) -> (w126:T2)
          n49 = Add(x=w99, y=w96) -> (x+y=w98:T5)
          n50 = Bundle By Name(cluster=w100, "Rectangle"=w98) -> (w101:T2)
          n51 = call <vilib>:"Draw Flattened Pixmap.vi"("image data"=w126, "picture"=w129) -> ("new picture"=w107:picture)  [unwired: 7 in]
          n52 = Less Or Equal?(x=w88, y=w87) -> (x <= y?=w94:bool)
          n53 = Select(t=w93, s=w94, f=w90) -> (s? t:f=w91:i32)
          n54 = call <vilib>:"Draw Flattened Pixmap.vi"("image data"=w101, "picture"=w107) -> ("new picture"=w106:picture)  [unwired: 7 in]
        }
        "Picture" <- w85
        n55 = Bundle By Name(cluster=w77, "Rectangles"=w78, "VerticalRows"=w64) -> (w79:T3)
      }
      frame "", "Idle" {
        n56 = event shown="[0] \"Picture\": Mouse Up" {
          selector: _ -> [_ _ _ _ _ _ _]
          dyn-events: _ -> [_ _ _ _ _ _ _]
          timeout: _ -> [_ _ _ _ _ _ _]
          tunnel: ["CheckSrollPos" ("format string") "HideRing" ("format string") "Redraw" ("format string") w161 "Exit" ("format string") "CheckSrollPos" ("format string") "CheckSrollPos" ("format string")] -> w137
          tunnel: w136 -> [w138 w141 w148 w157 w179 w181 w183]
          tunnel: [w138 w141 w144 w159 w179 w181 w183] -> w135
          event "Picture": Mouse Up {
            n57 = event-data() -> ()  [unwired: 1 in, 1 out]
          }
          event "Ring": Mouse Leave {
            n58 = event-data() -> ()  [unwired: 1 in, 3 out]
          }
          event "Ring": Value Change {
            n59 = event-data() -> ()  [unwired: 1 in, 2 out]
            n60 = Unbundle By Name(w148) -> ("Selected"=w147:i32[], "Row"=w146:i32)
            n61 = in-place {
              in-place-border: "Ring" -> [w149]
              n62 = in-place-array #1(w147, w146) -> ()  [unwired: 1 out]
              n63 = in-place-array #1(w149) -> (w143:i32[])  [unwired: 1 out]
            }
            n64 = Bundle By Name(cluster=w148, "Selected"=w143) -> (w144:T3)
          }
          event "Picture": Mouse Move {
            n65 = event-data() -> ()  [unwired: 1 in, 1 out]
            n66 = Unbundle By Name(w157) -> ("ShowRing"=w160:bool)
            n67 = property on="Picture" class="Pict"() -> ("Mouse"=w163:T9)  [unwired: 2 in, 2 out]
            n68 = Unbundle By Name(w163) -> ("Mouse Position"=w162:cluster{"X":i32, "Y":i32})
            "Mouse Position" <- w162
            n69 = Unbundle By Name(w157) -> ("IndexOffset"=w156:i32, "VerticalRows"=w150:i32, "Rectangles"=w151:T10)
            n70 = for {
              tunnel: w151 -> [w174] mode=indexing
              tunnel: w162 -> [w176]
              tunnel: [w175] -> w164
              tunnel: [w174] -> w158
              tunnel: [w173] -> w154
              i -> [w173]
              stop <- w175 stop-if-true
              n71 = call <vilib>:"PointInRect.vi"("rect"=w174, "point"=w176) -> ("pt in rect"=w175:bool)
            }
            n72 = Add(x=w156, y=w150) -> (x+y=w155:i32)
            n73 = Decrement(x=w155) -> (x-1=w153:i32)
            n74 = Less Or Equal?(x=w154, y=w153) -> (x <= y?=w152:bool)
            n75 = Compound Arithmetic op=AND(w152, w164, invert w160) -> (w165:bool)
            n76 = case shown="False" w165 {
              tunnel: w158 -> [_ _]
              tunnel: w164 -> [w169 _]
              tunnel: w160 -> [w167 _]
              tunnel: [w166 "ShowRing" ("format string")] -> w161
              frame False {
                n77 = Compound Arithmetic op=AND(invert w169, w167) -> (w168:bool)
                n78 = case shown="False" w168 {
                  tunnel: ["Idle" ("format string") "HideRing" ("format string")] -> w166
                  frame False {
                  }
                  frame True {
                  }
                }
              }
              frame True {
              }
            }
            n79 = Bundle By Name(cluster=w157, "Row"=w154, "Rectangle"=w158) -> (w159:T3)
          }
          event Panel Close? {
            n80 = event-data() -> ()  [unwired: 1 in, 1 out]
            n81 = event-data("Discard?"=TRUE) -> ()  [unwired: 1 in, 1 out]
          }
          event "Picture": Mouse Down {
            n82 = event-data() -> ()  [unwired: 1 in, 1 out]
          }
          event "Picture": Mouse Leave {
            n83 = event-data() -> ()  [unwired: 1 in, 1 out]
          }
        }
      }
      frame "CheckSrollPos" {
        n84 = property on="Picture" class="Pict"() -> ("Top"=w184:i16)  [unwired: 2 in, 2 out]
        n85 = feedback-in #2(w184) -> ()
        n86 = feedback #2(i16 0 ("Top")) -> (w189:i16)
        n87 = Unbundle By Name(w192) -> ("Y-Distance"=w186:i32)  [unwired: 1 out]
        n88 = Subtract(x=w189, y=w184) -> (x-y=w188:i16)
        n89 = Sign(1:w188) -> (0:w187:i16)
        n90 = case shown="0, Default" w187 {
          tunnel: w184 -> [w203 w206 w207]
          tunnel: w186 -> [w202 w205 _]
          tunnel: [w201 w204 w207] -> _
          frame 1 {
            n91 = Subtract(x=w203, y=w202) -> (x-y=w201:i32)
          }
          frame -1 {
            n92 = Add(x=w206, y=w205) -> (x+y=w204:i32)
          }
          frame 0, Default {
          }
        }
        n93 = Quotient & Remainder(x=w184, y=w186) -> (x-y*floor(x/y)=w198:i32, floor(x/y)=w195:i32)
        n94 = Divide(x=w186, y=2) -> (x/y=w197:dbl)
        n95 = Greater Or Equal?(x=w198, y=w197) -> (x >= y?=w196:bool)
        n96 = Increment(x=w195) -> (x+1=w194:i32)
        n97 = Select(t=w194, s=w196, f=w195) -> (s? t:f=w193:i32)
        n98 = Multiply(x=w193, y=w186) -> (x*y=w200:i32)
        n99 = property on="Picture" class="Pict"("Top"=w200) -> ()  [unwired: 2 in, 2 out]
        n100 = Bundle By Name(cluster=w192, "IndexOffset"=w193) -> (w191:T3)
      }
      frame "ShowRing" {
        n101 = property on="Picture" class="Pict"() -> ("Draw Area Size"=w223:T6)  [unwired: 2 in, 2 out]
        n102 = Unbundle By Name(w229) -> ("YStart"=w210:i32, "Rectangle"=w234:T5, "IndexOffset"=w233:i32, "Y-Distance"=w224:i32, "XStart2"=w219:i32)
        n103 = Unbundle By Name(w229) -> ("Row"=w214:i32, "Selected"=w215:i32[])
        n104 = Unbundle By Name(w223) -> ("Width"=w222:u32)
        n105 = Index Array(array=w227, index=w214) -> (element=w226:T11)
        n106 = Index Array(array=w215, index=w214) -> (element=w213:i32)
        n107 = Add(x=w222, y=u32 3) -> (x+y=w220:u32)
        n108 = Subtract(x=w220, y=w219) -> (x-y=w217:u32)
        n109 = Unbundle By Name(w226) -> ("Options"=w225:string[])
        n110 = Unbundle By Name(w234) -> ("left"=w241:i16, "top"=w239:i16)
        n111 = property on="Picture" class="Pict"() -> ("MasterRect"=w243:T12)  [unwired: 2 in, 2 out]
        n112 = Multiply(x=w233, y=w224) -> (x*y=w231:i32)
        n113 = Unbundle By Name(w243) -> ("Left"=w242:i16, "Top"=w240:i16)
        n114 = Bundle(cluster=T6 {"Width"=93, "Height"=17} ("Named Numeric Size"), "Width"=w217) -> (w216:T6)  [unwired: 1 in]
        n115 = Add(x=w242, y=w241) -> (x+y=w230:i16)
        n116 = Add(x=w240, y=w239) -> (x+y=w232:i16)
        n117 = Subtract(x=w210, y=2 ("x")) -> (x-y=w209:i32)
        n118 = Decrement(x=w230) -> (x-1=w228:i16)
        n119 = Subtract(x=w232, y=w231) -> (x-y=w212:i32)
        n120 = Add(x=w212, y=w209) -> (x+y=w211:i32)
        n121 = Bundle By Name(cluster=w229, "ShowRing"=TRUE) -> (w238:T3)
        n122 = property on="Ring" class="Ring (strict)"("Strings []"=w225, "Value"=w213, "Left"=w228, "Top"=w211, "NmdNumSize"=w216, "Visible"=TRUE ("ShowRing")) -> ()  [unwired: 2 in, 2 out]
      }
      frame "HideRing" {
        n123 = Bundle By Name(cluster=w248, "ShowRing"=FALSE) -> (w247:T3)
        n124 = property on="Ring" class="Ring (strict)"("Visible"=FALSE ("ShowRing")) -> ()  [unwired: 2 in, 2 out]
      }
      frame Default {
      }
    }
    n125 = Equal?(x=w14, y="Exit" ("format string")) -> (x = y?=w12:bool)
  }
  n126 = stacked-sequence {
    tunnel: w5 -> [_]
    frame #0 {
      n127 = property on="Picture" class="Pict"() -> ("Left"=w255:i32, "Top"=w254:i32)  [unwired: 2 in, 2 out]
      n128 = Subtract(x=w254, y=25 ("x")) -> (x-y=w253:i32)
      n129 = property on="Ring" class="Ring (strict)"("Left"=w255, "Top"=w253, "Visible"=TRUE) -> ()  [unwired: 2 in, 2 out]
    }
  }
